vi "Get ni_bus_monitor_api_LastCommError.vi"(8 "error in (no error)":errorcluster, 11 "gRPCid":T1) -> (0 "error out":errorcluster, 2 "package_template_enum":T2, 3 "gRPCid out":T1)   [LabVIEW 2025, in "bus_monitor_server.lvlib"]
uses:
  bus_monitor_server.lvlib
  ni_bus_monitor_api_LastCommError.ctl
  <vilib>/gRPC/LabVIEW gRPC Library/Shared/grpcId.ctl
  2ed25e12-861d-4677-8ead-ace2906b2041.vi
  <vilib>/gRPC/LabVIEW gRPC Library/Shared/TranslateGrpcError.vi
  <vilib>/gRPC/LabVIEW gRPC Library/Server API/Server/Get Server DLL Path.vi
  <vilib>/Utility/error.llb/Error Cluster From Error Code.vi
  <vilib>/gRPC/LabVIEW gRPC Library/grpc-lvsupport-release.lvlib
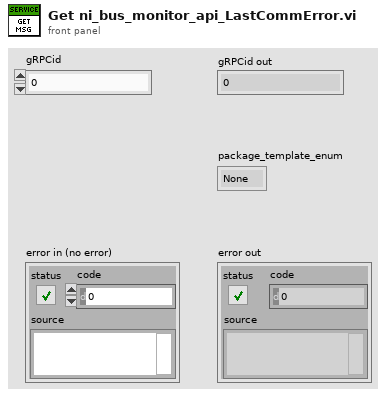
[diagram p1: front panel]
types:
  T1 = typedef "grpc-lvsupport-release.lvlib/grpcId.ctl" = u64
  T2 = typedef "bus_monitor_server.lvlib/ni_bus_monitor_api_LastCommError.ctl" = enum32{"None", "Stuff", "Form", "ACK", "Bit1", "Bit0", "CRC"}
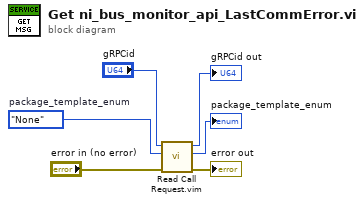
[diagram p0: block diagram]
diagram:
  w2 = ni_bus_monitor_api_LastCommError."None"  # package_template_enum
  n1 = call "Read Call Request.vim"("error in"="error in (no error)", "Request Type"=w2, "gRPCid in"="gRPCid") -> ("error out"=→"error out":errorcluster, "Request Data"=→"package_template_enum":T2, "gRPCid out"=→"gRPCid out":T1)  [unwired: 6 in]
